vi "inputsChartView.vi"(10 "UserEvents in":refnum<class "UserEvents.lvclass">) -> ()   [LabVIEW 2015, in "M1M3SSSTViews.lvlib"]
uses:
  M1M3SSSTViews.lvlib
  UserEvents/UserEvents.lvclass
  UserEvents/UserEvents.lvclass/UserEvents.ctl
  Typedefs/StateSelector.ctl
  Typedefs/M1M3SSSTypedefs.lvlib
panel:
  out "Force vs. Time":dbl(graph)
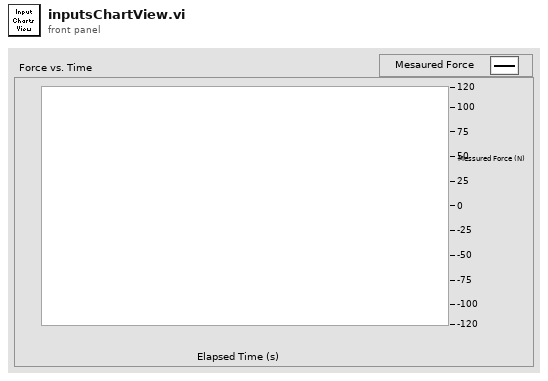
[diagram p1: front panel]
types:
  T1 = typedef "M1M3SSSTypedefs.lvlib/PubDataEvents.ctl" = cluster{"State":refnum<user-event>, "ErrorCode":refnum<user-event>, "OutputData":refnum<user-event>, "InputData":refnum<user-event>, "ControllerData":refnum<user-event>, "TestStatus":refnum<user-event>, "LogPath":refnum<user-event>, "StiffnessData":refnum<user-event>}
  T2 = cluster{"Event Registration Refnum":refnum<event-registration>, "Event Registration Refnum":refnum<event-registration>}
  T3 = typedef "M1M3SSSTypedefs.lvlib/StateSelector.ctl" = enum16{"FaultState", "OffState", "RampingUpPressurePState", "RampingUpPressureSTState", "StandbyState", "StoppedState", "WaitingForSettledPState", "WaitingForSettledSTState"}
  T4 = typedef "M1M3SSSTypedefs.lvlib/ForceDemand.ctl" = dbl[unit]
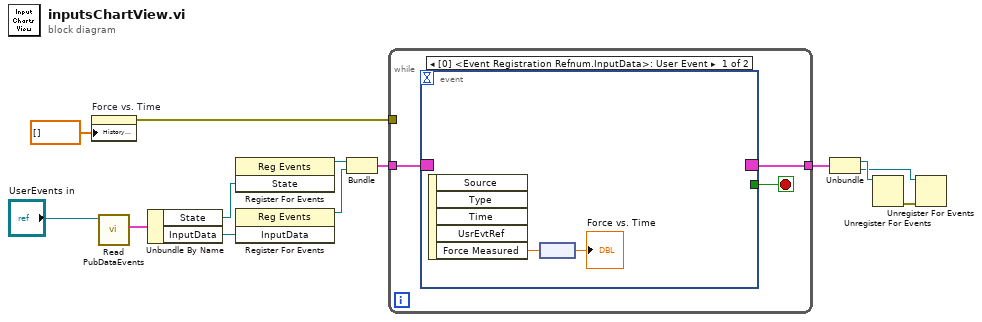
[diagram p0: block diagram]
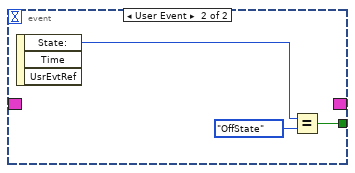
[diagram p2: hidden frame]
diagram:
  n1 = property on="Force vs. Time" class="WFChart (strict)"("History Data"=dbl[] []) -> (error out=w3:errorcluster)  [unwired: 2 in, 1 out]
  n2 = call "Read PubDataEvents.vi"("UserEvents in"="UserEvents in") -> ("PubDataEvents"=w13:T1)  [unwired: 9 in, 1 out]
  n3 = Unbundle By Name(w13) -> ("State"=w12:refnum<user-event>, "InputData"=w10:refnum<user-event>)
  n4 = register-events(w12) -> (reference out=w11:refnum<event-registration>)  [unwired: 2 in, 1 out]
  n5 = register-events(w10) -> (reference out=w9:refnum<event-registration>)  [unwired: 2 in, 1 out]
  n6 = Bundle("Event Registration Refnum"=w11, "Event Registration Refnum"=w9) -> (w7:T2)  [unwired: 1 in]
  n7 = while {
    tunnel: w7 -> [w14]
    tunnel: w3 -> [_]
    tunnel: [w15] -> w1
    stop <- w16 stop-if-true
    n8 = event shown="[0] <Event Registration Refnum.InputData>: User Event" {
      selector: w14 -> [_ _]
      dyn-events: [_ _] -> w15
      timeout: _ -> [_ _]
      tunnel: [_ w20] -> w16
      event User Event {
        n9 = event-data() -> ("Force Measured"=w18:T4)  [unwired: 1 in, 4 out]
        n10 = node(w18) -> (→"Force vs. Time":dbl)
      }
      event User Event {
        n11 = event-data() -> ("State:"=w19:T3)  [unwired: 1 in, 2 out]
        n12 = Equal?(x=w19, y=StateSelector."OffState" ("State:")) -> (x = y?=w20:bool)
      }
    }
  }
  n13 = Unbundle(w1) -> ("Event Registration Refnum"=w6:refnum<event-registration>, "Event Registration Refnum"=w5:refnum<event-registration>)
  n14 = Unregister For Events(event registration refnum=w6) -> (error out=w4:errorcluster)  [unwired: 1 in]
  n15 = Unregister For Events(event registration refnum=w5, error in=w4) -> ()  [unwired: 1 out]
